vi "Destroy.vi"(8 "error in (no error)":errorcluster, 10 "Wait for Stop Timeout ms (-1)":i32=-1, 11 "API-Reference in":refnum<k1>) -> (0 "error out":errorcluster, 1 "Timeout":bool, 3 "Final State":refnum<class "Copy of Actor.lvclass">)   [LabVIEW 2018, in "Copy of Actor.lvclass"]
uses:
  Copy of Actor.lvclass
  API-Data.ctl
  Stopped.ctl
  Event-References.ctl
  Stop.ctl
  Launched.ctl
  Some Request.ctl
  Some Response.ctl
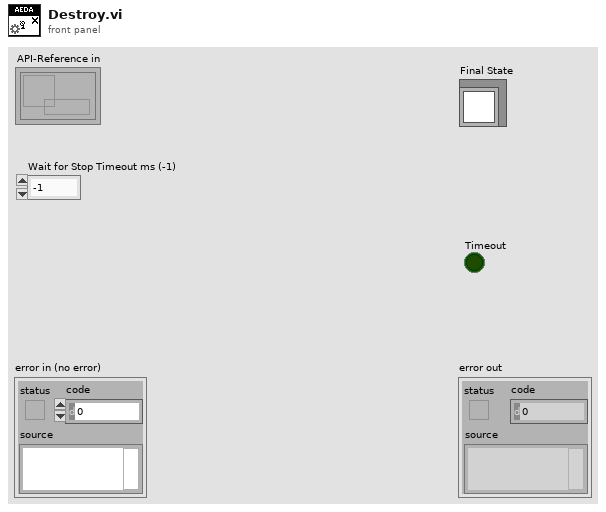
[diagram p1: front panel]
types:
  T1 = typedef "Copy of Actor.lvclass/API-Data.ctl" = cluster{"Launch":refnum<notifier>, "Stopped":refnum<user-event>, "Actor-Events":T2, "Stopped Registration":refnum<event-registration>}
  T2 = typedef "Copy of Actor.lvclass/Event-References.ctl" = cluster{"Stop":refnum<user-event>, "Launched":refnum<user-event>, "Some Request":refnum<user-event>}
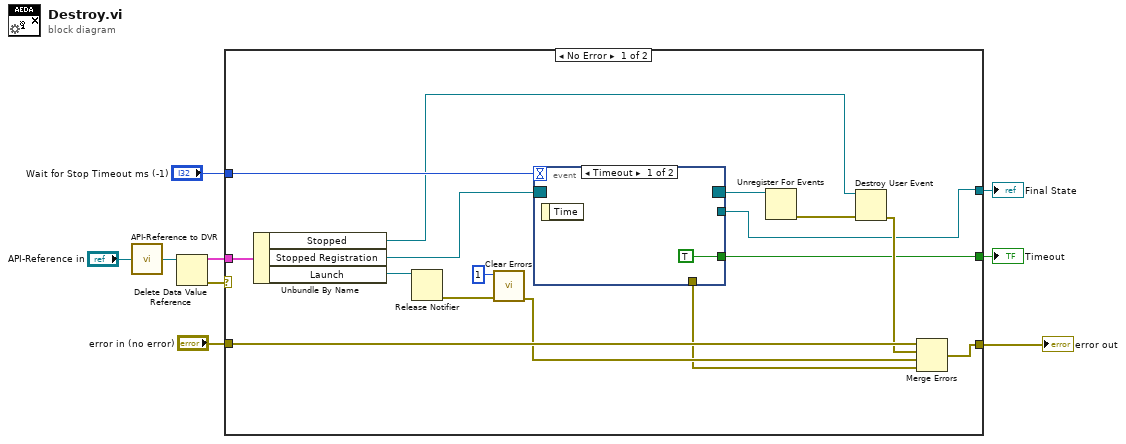
[diagram p0: block diagram]
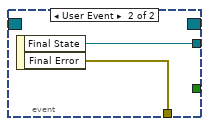
[diagram p2: hidden frame]
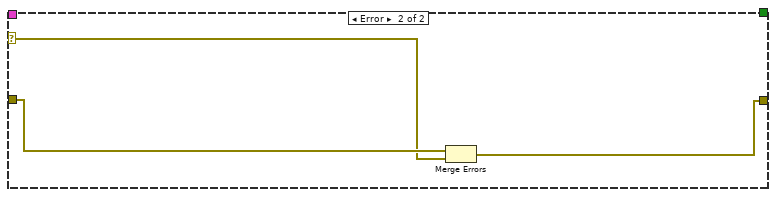
[diagram p3: hidden frame]
diagram:
  n1 = call "API-Reference to DVR.vi"("API-Reference in"="API-Reference in") -> ("Data Value Reference out"=w1:refnum<data-value>)
  n2 = Delete Data Value Reference(data value reference=w1) -> (data value=w9:T1, error out=w5:errorcluster)  [unwired: 1 in]
  n3 = case shown="No Error" w5 {
    selector: w5 -> [_ w30]
    tunnel: w9 -> [w25 _]
    tunnel: "error in (no error)" -> [w24 w31]
    tunnel: "Wait for Stop Timeout ms (-1)" -> [w20 _]
    tunnel: [w19 w29] -> w6
    tunnel: [w11 _] -> w4
    tunnel: [w10 _] -> w3
    frame No Error {
      n4 = Unbundle By Name(w25) -> ("Stopped"=w15:refnum<user-event>, "Stopped Registration"=w21:refnum<event-registration>, "Launch"=w18:refnum<notifier>)
      n5 = Release Notifier(notifier=w18) -> (error out=w17:errorcluster)  [unwired: 2 in, 2 out]
      n6 = call <vilib>:"Clear Errors.vi"("error in (no error)"=w17, "specific error code to clear (0: all)"=1) -> ("error out"=w23:errorcluster)  [unwired: 4 in, 1 out]
      n7 = event shown="[0] Timeout" {
        selector: w21 -> [_ _]
        dyn-events: [_ _] -> w13
        timeout: w20 -> [_ _]
        tunnel: [_ w28] -> w12
        tunnel: [TRUE _] -> w11
        tunnel: [_ w27] -> w10
        event Timeout {
          n8 = event-data() -> ()  [unwired: 1 in, 1 out]
        }
        event User Event {
          n9 = event-data() -> ("Final State"=w27:refnum<class "Copy of Actor.lvclass">, "Final Error"=w28:errorcluster)  [unwired: 1 in]
        }
      }
      n10 = Unregister For Events(event registration refnum=w13) -> (error out=w16:errorcluster)  [unwired: 1 in]
      n11 = Destroy User Event(user event=w15, error in=w16) -> (error out=w14:errorcluster)
      n12 = Merge Errors(w24, w14, w23, w12) -> (w19:errorcluster)
    }
    frame Error {
      n13 = Merge Errors(w31, w30) -> (w29:errorcluster)
    }
  }
  "error out" <- w6
  "Timeout" <- w4
  "Final State" <- w3
